vi "Test Set Symbol.vi"(8 "error in (no error)":errorcluster, 11 "Test Case In":refnum<class "Conditional Disabled Configurator Test.lvclass">) -> (0 "error out":errorcluster, 3 "Test Case Out":refnum<class "Conditional Disabled Configurator Test.lvclass">)   [LabVIEW 2020]
uses:
  01074fa8-ee8a-411d-bc8b-fc92c4f90959.vi
  test/Conditional Disabled Configurator Test/Conditional Disabled Configurator Test.lvclass
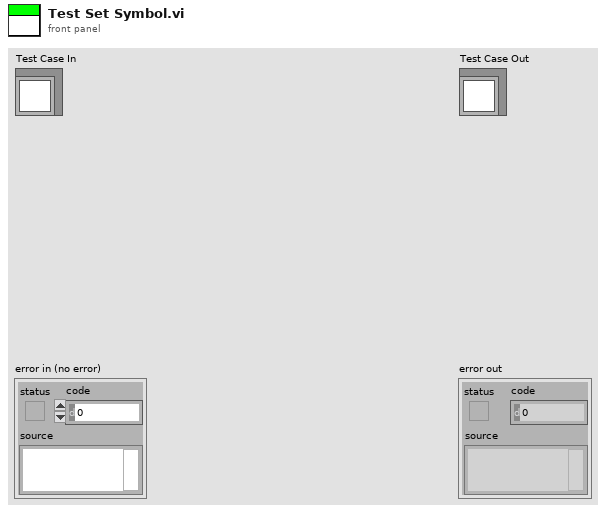
[diagram p1: front panel]
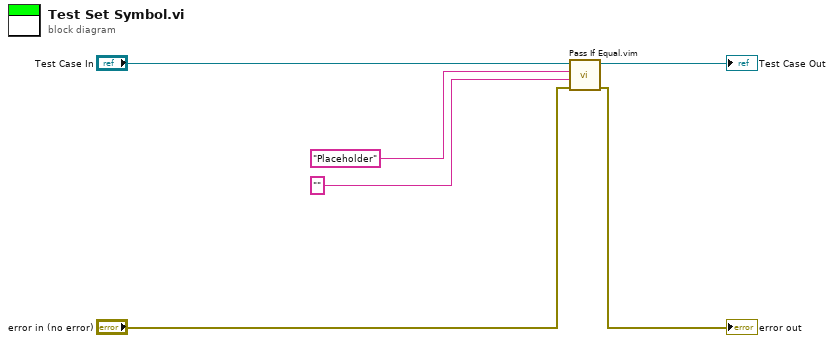
[diagram p0: block diagram]
diagram:
  n1 = call "Pass If Equal.vim"("error in (no error)"="error in (no error)", "Actual"="", "Expected"="Placeholder", "LUnit Test Case In"="Test Case In") -> ("error out"=→"error out":errorcluster, "LUnit Test Case Out"=→"Test Case Out":refnum<class "Conditional Disabled Configurator Test.lvclass">)  [unwired: 6 in]
